vi "Read targetRange.vi"(8 "error in (no error)":errorcluster, 11 "KickTactic in":refnum<class "KickTactic.lvclass">) -> (0 "error out":errorcluster, 2 "targetRange":dbl[](array[numeric]), 3 "KickTactic out":refnum<class "KickTactic.lvclass">)   [LabVIEW 2023, in "KickTactic.lvclass"]
uses:
  KickTactic.lvclass
  KickTactic.lvclass/KickTactic.ctl
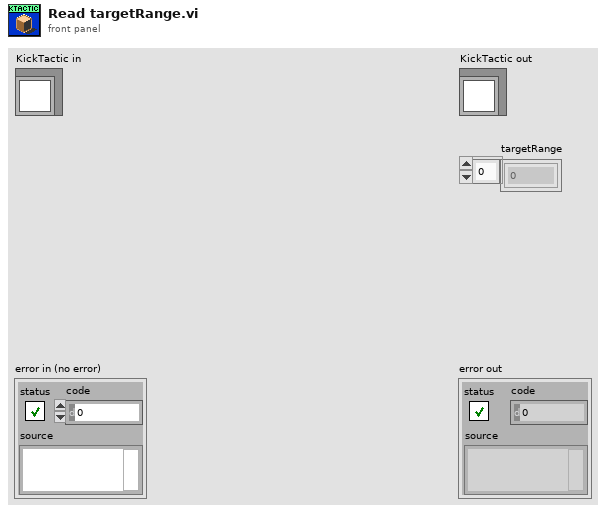
[diagram p1: front panel]
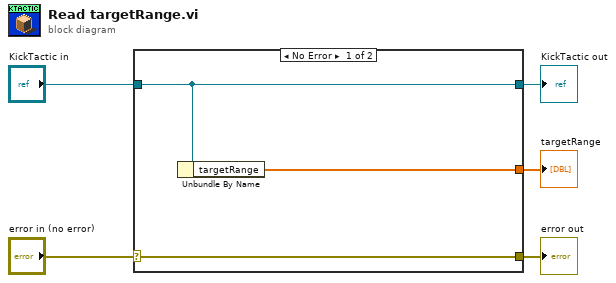
[diagram p0: block diagram]
diagram:
  n1 = case shown="No Error" "error in (no error)" {
    selector: "error in (no error)" -> [w8 w9]
    tunnel: [w8 w9] -> w4
    tunnel: [w7 w10] -> w2
    tunnel: "KickTactic in" -> [w7 w10]
    tunnel: [w6 _] -> w1
    frame No Error {
      n2 = Unbundle By Name(w7) -> ("targetRange"=w6:dbl[])
    }
    frame Error {
    }
  }
  "error out" <- w4
  "KickTactic out" <- w2
  "targetRange" <- w1
